vi "picoharp_read_fifo.vi"(8 "error in (no error)":errorcluster, 11 "hydraharp in":refnum<class "picoharp.lvclass">) -> (0 "error out":errorcluster, 2 "stop":bool, 3 "hydraharp out":refnum<class "picoharp.lvclass">)   [LabVIEW 2015, in "picoharp.lvclass"]
uses:
  picoharp.lvclass
  picoharp.lvclass/picoharp.ctl
  Hydraharp/hydraharp/hydraharp_fifo_queue_data.ctl
  Hydraharp/hydraharp/hydraharp_fifo_actions.ctl
  stop_pico_acq.vi
  phlib.dll
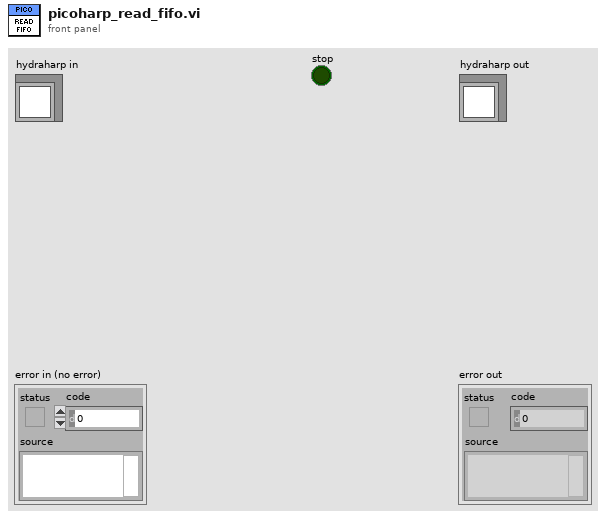
[diagram p1: front panel]
types:
  T1 = typedef "hydraharp_fifo_queue_data.ctl" = cluster{"fifo_buffer":u32[], "fifo_action":T2}
  T2 = typedef "hydraharp_fifo_actions.ctl" = enum16{"stop", "new_data"}
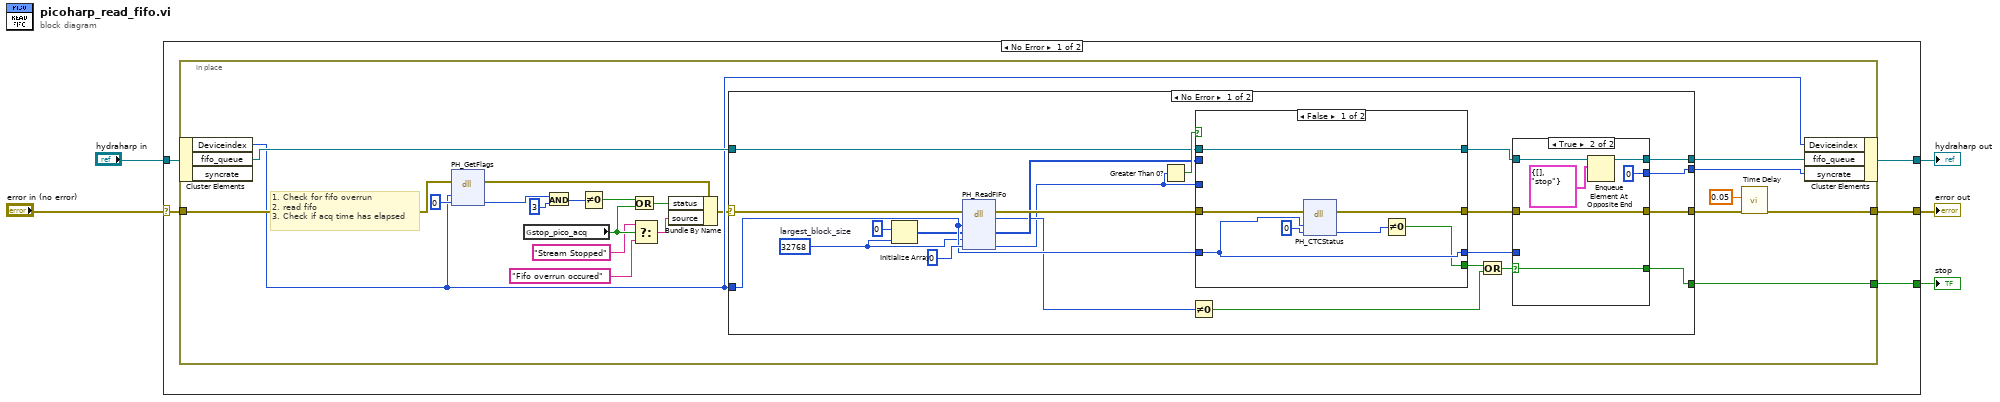
[diagram p0: block diagram]
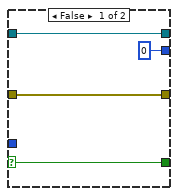
[diagram p2: hidden frame]
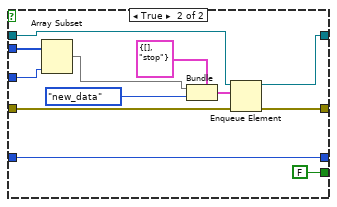
[diagram p3: hidden frame]
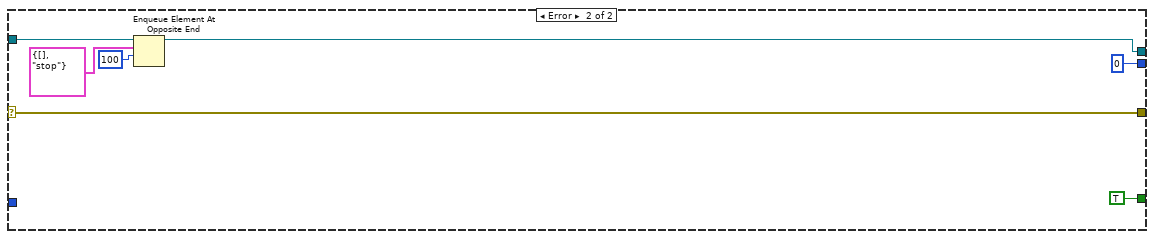
[diagram p4: hidden frame]
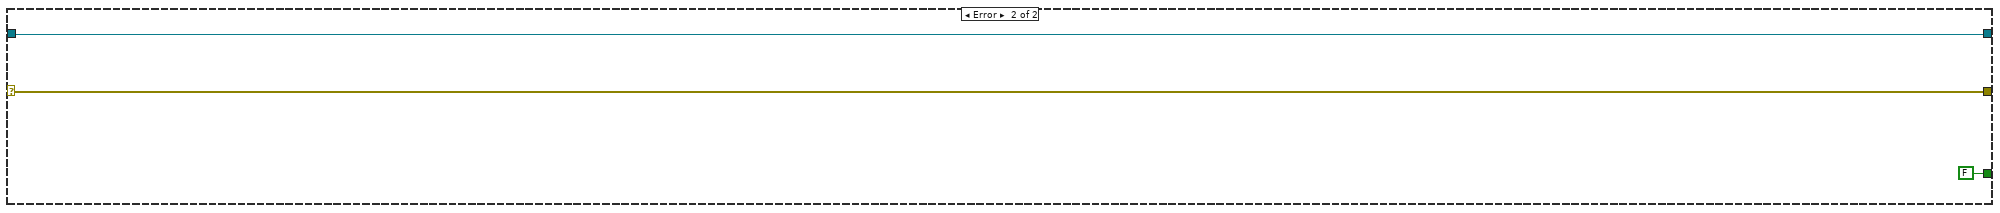
[diagram p5: hidden frame]
diagram:
  n1 = case shown="No Error" "error in (no error)" {
    selector: "error in (no error)" -> [w9 w92]
    tunnel: [w8 w92] -> w4
    tunnel: [w7 w91] -> w2
    tunnel: "hydraharp in" -> [w10 w91]
    tunnel: [w6 FALSE] -> w1
    frame No Error {
      n2 = in-place {
        in-place-border: w9 -> [w31]
        in-place-border: [w18] -> w8
        in-place-border: [w24] -> w6
        # "1. Check for fifo overrun\n2. read fifo\n3. Check if acq time has elapsed"
        n3 = in-place-cluster #1(w10) -> ("Deviceindex"=w25:i32, "fifo_queue"=w27:refnum<queue>)  [unwired: 1 out]
        n4 = dll-call lib="phlib.dll" fn="PH_GetFlags" label="pH_GetFlags"(error in=w31, "devidx"=w25, "flags"=0) -> (error out=w23:errorcluster, "flags"=w29:i32)  [unwired: 4 in, 1 out]
        n5 = global read "stop_pico_acq.vi" "stop_pico_acq"() -> (w13:bool)
        n6 = And(x=w29, y=3) -> (x .and. y?=w21:i32)
        n7 = Not Equal To 0?(x=w21) -> (x != 0?=w16:bool)
        n8 = Or(x=w16, y=w13) -> (x .or. y?=w15:bool)
        n9 = Select(t="Stream Stopped", s=w13, f="Fifo overrun occured" ("source")) -> (s? t:f=w11:string)
        n10 = Bundle By Name(cluster=w23, "status"=w15, "source"=w11) -> (w22:errorcluster)
        n11 = case shown="No Error" w22 {
          selector: w22 -> [w41 w85]
          tunnel: w25 -> [w50 _]
          tunnel: w27 -> [w48 w89]
          tunnel: [w44 w88] -> w26
          tunnel: [w43 w85] -> w19
          tunnel: [w42 TRUE] -> w24
          tunnel: [w32 0 ("syncrate")] -> w17
          frame No Error {
            w35 = 32768  # largest_block_size
            n12 = Initialize Array(u32 0 ("element"), w35) -> (w34:u32[])
            n13 = dll-call lib="phlib.dll" fn="PH_ReadFiFo" label="pH_ReadFiFo"(error in=w41, "devidx"=w50, "buffer"=w34, "blocksize"=w35, "nactual"=0) -> (error out=w51:errorcluster, "return type"=w40:i32, "buffer"=w47:u32[], "nactual"=w37:i32)  [unwired: 4 in, 1 out]
            n14 = Greater Than 0?(x=w37) -> (x > 0?=w52:bool)
            n15 = Not Equal To 0?(x=w40) -> (x != 0?=w39:bool)
            n16 = case shown="False" w52 {
              tunnel: w51 -> [w70 w80]
              tunnel: [w69 w75] -> w38
              tunnel: w50 -> [w67 w71]
              tunnel: [w64 FALSE] -> w49
              tunnel: w48 -> [w68 w81]
              tunnel: w47 -> [_ w74]
              tunnel: [w68 w76] -> w45
              tunnel: w37 -> [_ w72]
              tunnel: [w67 w71] -> w33
              frame False {
                n17 = dll-call lib="phlib.dll" fn="PH_CTCStatus" label="pH_CTCStatus"(error in=w70, "devidx"=w67, "status"=0) -> (error out=w69:errorcluster, "status"=w65:i32)  [unwired: 4 in, 1 out]
                n18 = Not Equal To 0?(x=w65) -> (x != 0?=w64:bool)
              }
              frame True {
                n19 = Array Subset(array=w74, length=w72) -> (w73:u32[])  [unwired: 1 in]
                n20 = Bundle(cluster=T1 {"fifo_buffer"=[], "fifo_action"=enum."stop"} ("output cluster"), "fifo_buffer"=w73, "fifo_action"=hydraharp_fifo_actions."new_data") -> (w77:T1)
                n21 = Enqueue Element(queue=w81, element=w77, error in (no error)=w80) -> (queue out=w76:refnum<queue>, error out=w75:errorcluster)  [unwired: 1 in, 1 out]
              }
            }
            n22 = Or(x=w49, y=w39) -> (x .or. y?=w46:bool)
            n23 = case shown="True" w46 {
              selector: w46 -> [w55 w60]
              tunnel: w45 -> [w57 w63]
              tunnel: [w57 w61] -> w44
              tunnel: w38 -> [w56 w59]
              tunnel: [w56 w59] -> w43
              tunnel: [w55 w60] -> w42
              tunnel: w33 -> [_ _]
              tunnel: [0 ("syncrate") 0 ("syncrate")] -> w32
              frame False {
              }
              frame True {
                n24 = Enqueue Element At Opposite End(queue=w63, element=T1 {"fifo_buffer"=[], "fifo_action"=enum."stop"}) -> (queue out=w61:refnum<queue>)  [unwired: 2 in, 2 out]
              }
            }
          }
          frame Error {
            n25 = Enqueue Element At Opposite End(queue=w89, element=T1 {"fifo_buffer"=[], "fifo_action"=enum."stop"}, timeout in ms (-1)=100) -> (queue out=w88:refnum<queue>)  [unwired: 1 in, 2 out]
          }
        }
        n26 = call "Time Delay"("error in (no error)"=w19, "Delay Time (s)"=0.05) -> ("error out"=w18:errorcluster)  [unwired: 9 in]
        n27 = in-place-cluster #1("Deviceindex"=w25, "fifo_queue"=w26, "syncrate"=w17) -> (w7:refnum<class "picoharp.lvclass">)
      }
    }
    frame Error {
    }
  }
  "error out" <- w4
  "hydraharp out" <- w2
  "stop" <- w1
